vi "Main.vi"() -> ()   [LabVIEW 2017]
uses:
  ExperimentVariables.ctl
  AODControl/AODControlFiles/InterfaceReferences.ctl
  ImageAcquisitionProgram/ImageAcquisitionLibrary/References.ctl
  State.ctl
  SubVIQueues.ctl
  AODControl/MessageQueue/QueueOperations/All Message Queues.ctl
  AODControl/MessageQueue/QueueOperations/Message Cluster.ctl
  CircleControls.ctl
  <vilib>/Utility/error.llb/DialogType.ctl
  AODControl/AODGlobals.vi
  ImageAcquisitionProgram/ImageAcquisitionLibrary/GlobalFrontPanelReferences.vi
  MessageQueue/QueueOperations/Enqueue Message (Single).vi
  AODControl/AODControl.lvlib
  MessageQueue/MessageQueue.lvlib
  AODControl/MessageQueue/MessageQueue.lvlib
  ImageAcquisitionProgram/ImageAcquisitionLibrary/ImageAcquisitionLibrary.lvlib
panel:
  in  "Angle":dbl min=0.0 step=0.1 format="%#_6p"
  in  "Seq":bool
  in  "FlipY":bool
  in  "FlipX":bool
  in  "Phase":dbl step=0.1
  in  "Eccen.":dbl=1.0 min=0.0 step=0.05
  in  "Run":bool
  in  "Abort":bool
  in  "Script Path":path=path "D:/Dropbox/MyPrograms/LabViewLibraries/AODExperimentControls/ReologyScript.vi"
  in  "HexLatt":bool
  in  "Hold":bool
  in  "Hold":bool
  in  "Lattice Constant":dbl=10.0 step=0.05
  in  "Size":i32=1 min=1 step=1
  in  "PointSpec":enum32{"No. Of Points", "Density"}(radio)
  in  "No. of Points":i32=3 step=1
  in  "Exit":bool
  in  "Settings":T1={"Calibration Input"=[], "CalibrationResults"={"Center in Pixels"=[374.0120339529387, 375.46592887074246], "Angle"=0.022945275255000355, "Pixels/MHz X"=0.0, "Pixels/MHz Y"=0.0}, "Highlight"=[], "Running Script"=refnum}
  in  "Density":dbl=1.0 step=0.05
  in  "Center":cluster{"X":dbl, "Y":dbl}
  in  "Radius":dbl=10.0 step=0.05
  in  "Circle":bool
  in  "Exit Button":bool
  in  "Load":bool
  in  "Save":bool
  in  "Reset":bool
  out "Points":i32[][](array[numeric])
  in  "Calibrate":bool
  # "Draw an Ellipse"
  # "Draw a Hexagonal Lattice"
  # "Run a Script"
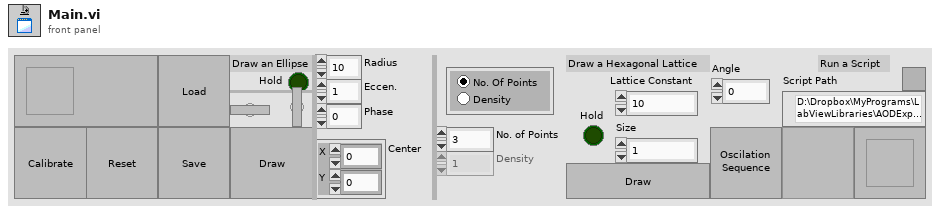
[diagram p1: front panel]
types:
  T1 = typedef "ExperimentVariables.ctl" = cluster{"Calibration Input":i32[][], "CalibrationResults":cluster{"Center in Pixels":dbl[], "Angle":dbl, "Pixels/MHz X":dbl, "Pixels/MHz Y":dbl}, "Highlight":i32[], "Running Script":refnum<vi>}
  T2 = typedef "SubVIQueues.ctl" = cluster{"AOD Queue":T3}
  T3 = typedef "AODControl.lvlib/MessageQueue.lvlib/All Message Queues.ctl" = cluster{" AOD Interface":refnum<queue>}
  T4 = typedef "State.ctl" = enum16{"Point", "Move", "Calibrating"}
  T5 = typedef "ExperimentControls" = cluster{"AOD Controls":T6, "ImageAcquisitionRefs":T7}
  T6 = typedef "AODControl.lvlib/InterfaceReferences.ctl" = cluster{"AOD Points Display":refnum<vi>, "AOD Array":refnum<vi>, "AOD Array Size":refnum<vi>, "Replace Array List":refnum<vi>, "Replace List":refnum<vi>, "Remove":refnum<vi>, "Index":refnum<vi>, "Move":refnum<vi>, "X":refnum<vi>, "Y":refnum<vi>, "Add":refnum<vi>, "Load":refnum<vi>, "Save":refnum<vi>, "Exit":refnum<vi>, "Dynamic":refnum<vi>, "Rotate":refnum<vi>, "Rotation Speed":refnum<vi>, "Scaling Speed":refnum<vi>, "X Trans Speed":refnum<vi>, "Y Trans Speed":refnum<vi>, "Movie Array":refnum<vi>}
  T7 = typedef "ImageAcquisitionLibrary.lvlib/References.ctl" = cluster{"Acquire":refnum<vi>, "Rec":refnum<vi>, "Tracking":refnum<vi>, "Settings":refnum<vi>, "Stop":refnum<vi>, "Initialized?":bool, "ImDisplay":refnum<vi>}
  T8 = typedef "MessageQueue.lvlib/All Message Queues.ctl" = cluster{" Interface":refnum<queue>, "Joystick":refnum<queue>}
  T9 = typedef "CircleControls.ctl" = cluster{"Radius":dbl, "No. of Points":i32, "Center":cluster{"X":dbl, "Y":dbl}, "Circle":bool, "Density":dbl, "PointSpec":enum32{"No. Of Points", "Density"}, "Hold":bool, "Size":i32, "LatC":dbl, "Eccentricity":dbl, "Phase":dbl}
  T10 = enum8{"Enabled", "Disabled", "Disabled and Grayed Out"}
  T11 = typedef "DialogType.ctl" = u16
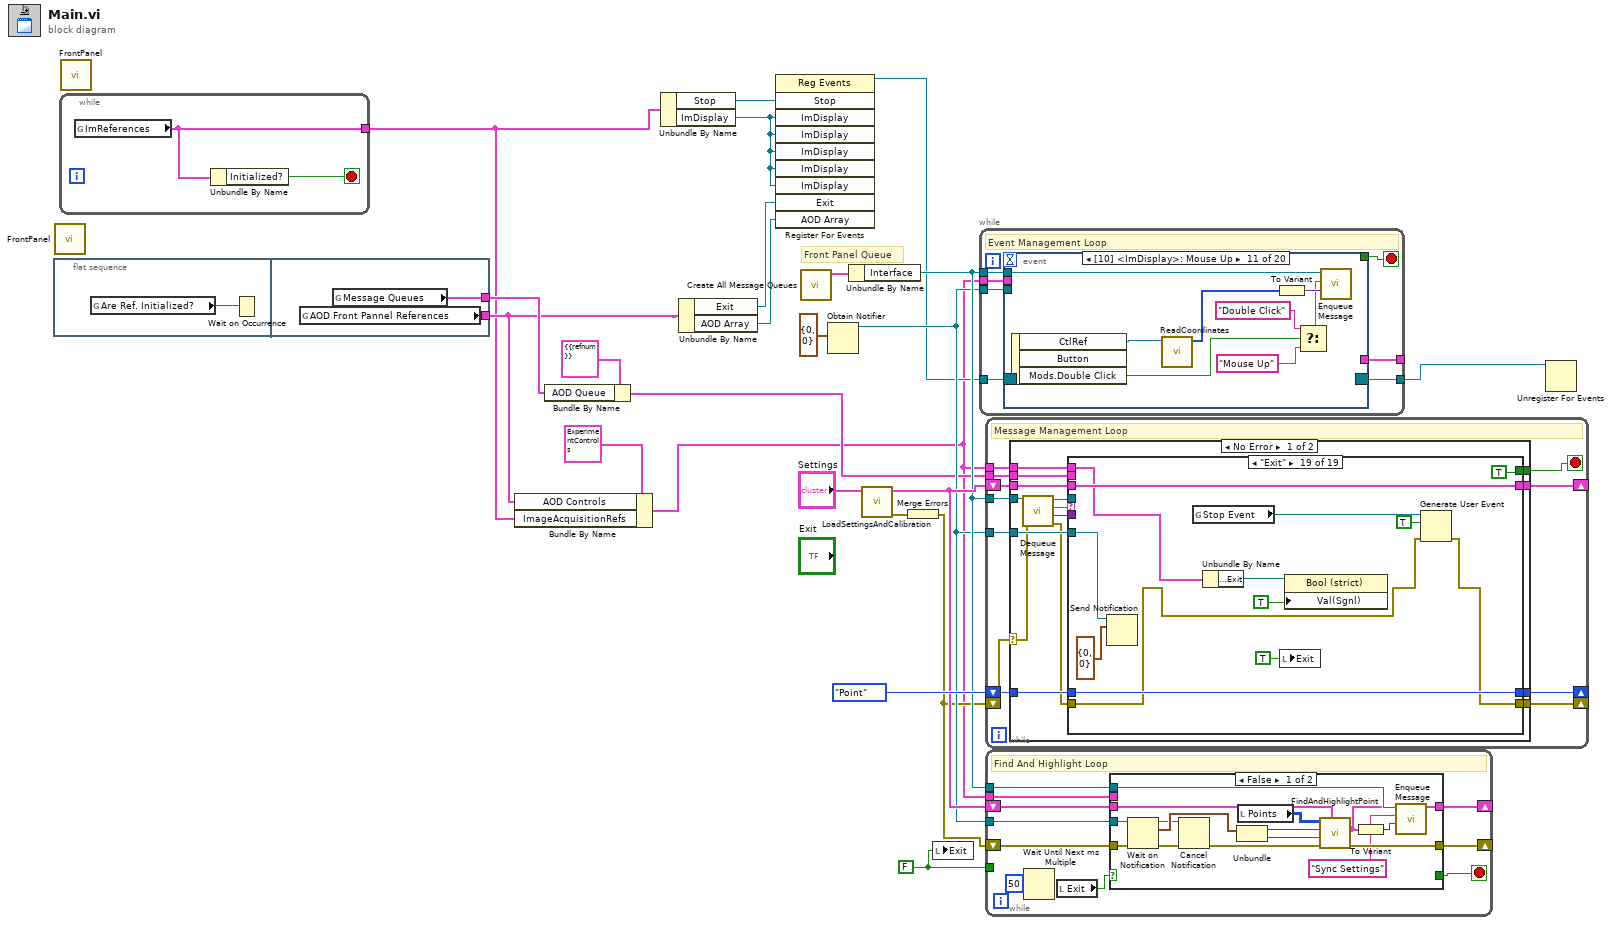
[diagram p0: block diagram]
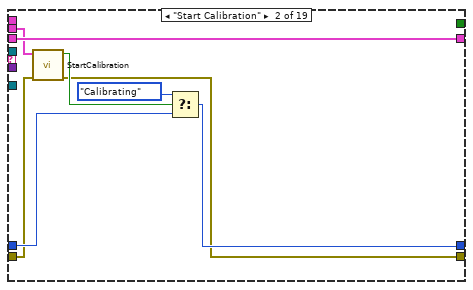
[diagram p4: hidden frame]
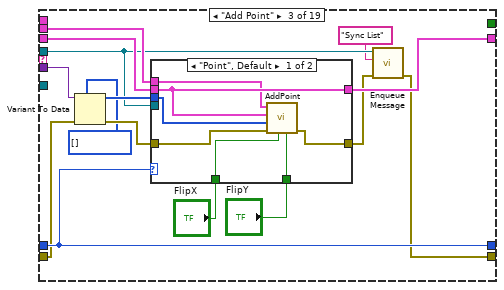
[diagram p5: hidden frame]
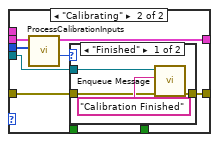
[diagram p6: hidden frame]
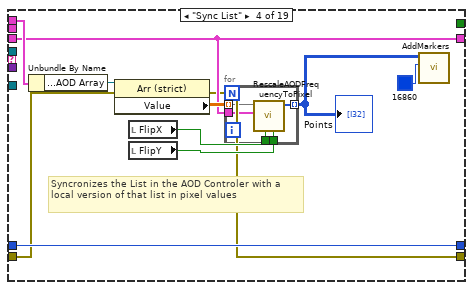
[diagram p8: hidden frame]
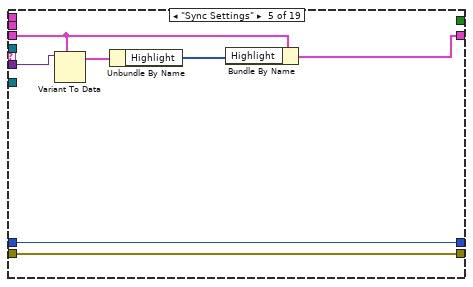
[diagram p9: hidden frame]
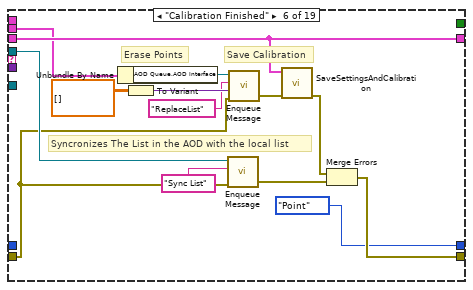
[diagram p10: hidden frame]
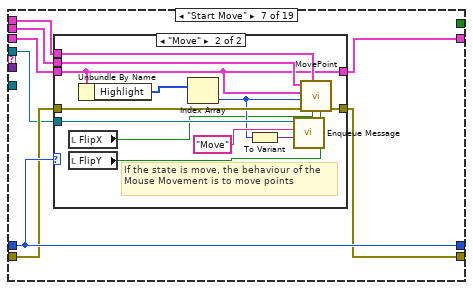
[diagram p11: hidden frame]
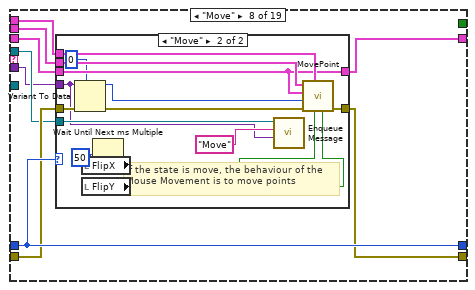
[diagram p13: hidden frame]
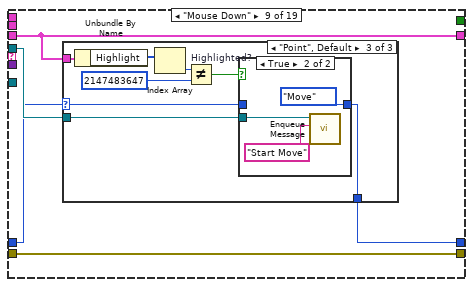
[diagram p15: hidden frame]
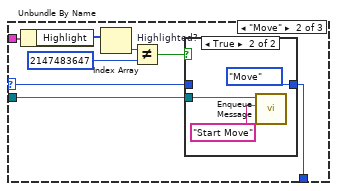
[diagram p17: hidden frame]
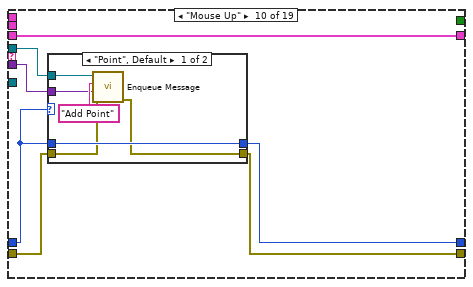
[diagram p20: hidden frame]
diagram:
  w17 = FALSE
  # "Front Panel Queue"
  n1 = flat-sequence {
    tunnel: [w26] -> w9
    tunnel: [w25] -> w6
    frame #0 {
      n2 = global read "AODGlobals.vi" "Are Ref. Initialized?"() -> (w24:refnum<k4>)
      n3 = Wait on Occurrence(2:w24) -> ()  [unwired: 2 in, 1 out]
    }
    frame #1 {
      n4 = global read "AODGlobals.vi" "AOD Front Pannel References"() -> (w25:T6)
      n5 = global read "AODGlobals.vi" "Message Queues"() -> (w26:T3)
    }
  }
  n6 = call "FrontPanel.vi"() -> ()  [unwired: 12 in]
  n7 = while {
    tunnel: [w27] -> w1
    stop <- w28 stop-if-true
    n8 = global read "GlobalFrontPanelReferences.vi" "ImReferences"() -> (w27:T7)
    n9 = Unbundle By Name(w27) -> ("Initialized?"=w28:bool)
  }
  n10 = call "FrontPanel.vi"() -> ()  [unwired: 12 in]
  n11 = Bundle By Name(cluster=T5 {"AOD Controls"={"AOD Points Display"=refnum, "AOD Array"=refnum, "AOD Array Size"=refnum, "Replace Array List"=refnum, "Replace List"=refnum, "Remove"=refnum, "Index"=refnum, "Move"=refnum, "X"=refnum, "Y"=refnum, "Add"=refnum, "Load"=refnum, "Save"=refnum, "Exit"=refnum, "Dynamic"=refnum, "Rotate"=refnum, "Rotation Speed"=refnum, "Scaling Speed"=refnum, "X Trans Speed"=refnum, "Y Trans Speed"=refnum, "Movie Array"=refnum}, "ImageAcquisitionRefs"={"Acquire"=refnum, "Rec"=refnum, "Tracking"=refnum, "Settings"=refnum, "Stop"=refnum, "Initialized?"=FALSE, "ImDisplay"=refnum}}, "AOD Controls"=w6, "ImageAcquisitionRefs"=w1) -> (w4:T5)
  n12 = Bundle By Name(cluster=T2 {"AOD Queue"={" AOD Interface"=refnum}} ("Queues Out"), "AOD Queue"=w9) -> (w10:T2)
  n13 = Unbundle By Name(w1) -> ("Stop"=w3:refnum<vi>, "ImDisplay"=w2:refnum<vi>)
  n14 = Unbundle By Name(w6) -> ("Exit"=w8:refnum<vi>, "AOD Array"=w7:refnum<vi>)
  n15 = register-events(w3, w2, w2, w2, w2, w2, w8, w7) -> (reference out=w12:refnum<event-registration>)  [unwired: 2 in, 1 out]
  n16 = call "Create All Message Queues.vi"() -> ("Message Queues out"=w23:T8)  [unwired: 10 in, 1 out]
  n17 = Obtain Notifier(notification data type=cluster{"X":i32, "Y":i32} {"X"=0, "Y"=0} ("Last Mouse Position:All Elements")) -> (notifier out=w14:refnum<notifier>)  [unwired: 3 in, 2 out]
  n18 = Unbundle By Name(w23) -> ("Interface"=w15:refnum<queue>)
  n19 = call "LoadSettingsAndCalibration.vi"("Cluster in"="Settings") -> ("error out"=w19:errorcluster, "Cluster out"=w16:T1)  [unwired: 9 in]
  n20 = Merge Errors(w19) -> (w13:errorcluster)
  n21 = local write "Exit"(w17) -> ()
  n22 = while {
    tunnel: w12 -> [w35]
    tunnel: w15 -> [w34]
    tunnel: w4 -> [w33]
    tunnel: [w32] -> w21
    tunnel: w14 -> [w30]
    tunnel: [w29] -> _
    stop <- w31 stop-if-true
    # "Event Management Loop"
    n23 = event shown="[10] <ImDisplay>: Mouse Up" {
      selector: w35 -> [_ _ _ _ _ _ _ _ _ _ _ _ w95 w96 _ _ _ _ _ _]
      dyn-events: [_ _ _ _ _ _ _ _ _ _ _ _ w94 w99 _ _ _ _ _ _] -> w32
      timeout: _ -> [_ _ _ _ _ _ _ _ _ _ _ _ _ _ _ _ _ _ _ _]
      tunnel: w34 -> [w36 w39 w43 w45 w47 w49 w63 w72 _ w81 w89 w91 _ _ _ w104 w107 w109 w111 w114]
      tunnel: w33 -> [_ _ _ _ _ _ _ _ _ _ _ _ w93 w98 _ _ _ _ _ _]
      tunnel: [TRUE TRUE _ _ _ _ _ _ _ _ _ _ _ _ _ _ _ _ TRUE TRUE] -> w31
      tunnel: w30 -> [_ _ _ _ _ _ _ _ _ _ _ _ _ _ w101 _ _ _ _ _]
      tunnel: [_ _ _ _ _ _ w60 w69 _ _ _ _ _ _ _ _ _ _ _ _] -> w29
      event Value Change {
        n24 = event-data() -> ()  [unwired: 1 in, 1 out]
        n25 = call-poly "Enqueue Message.vi"("Message"="Exit", "Message Queue"=w36) -> ()  [unwired: 8 in, 2 out]
      }
      event Value Change {
        n26 = event-data() -> ()  [unwired: 1 in, 1 out]
        n27 = call-poly "Enqueue Message.vi"("Message"="Exit", "Message Queue"=w39) -> ()  [unwired: 8 in, 2 out]
      }
      event "Calibrate": Value Change {
        n28 = event-data() -> ()  [unwired: 1 in, 1 out]
        n29 = call-poly "Enqueue Message.vi"("Message"="Start Calibration", "Message Queue"=w43) -> ()  [unwired: 8 in, 2 out]
      }
      event "Reset": Value Change {
        n30 = event-data() -> ()  [unwired: 1 in, 1 out]
        n31 = call-poly "Enqueue Message.vi"("Message"="Reset AOD", "Message Queue"=w45) -> ()  [unwired: 8 in, 2 out]
      }
      event "Save": Value Change {
        n32 = event-data() -> ()  [unwired: 1 in, 1 out]
        n33 = call-poly "Enqueue Message.vi"("Message"="Save List", "Message Queue"=w47) -> ()  [unwired: 8 in, 2 out]
      }
      event "Load": Value Change {
        n34 = event-data() -> ()  [unwired: 1 in, 1 out]
        n35 = call-poly "Enqueue Message.vi"("Message"="Load List", "Message Queue"=w49) -> ()  [unwired: 8 in, 2 out]
      }
      event "Circle", "Center", "Density", "Radius", "No. of Points", "Eccen.", "Phase": Value Change {
        n36 = event-data() -> ()  [unwired: 1 in, 1 out]
        n37 = Bundle(cluster=T9 {"Radius"=0.0, "No. of Points"=0, "Center"={"X"=0.0, "Y"=0.0}, "Circle"=FALSE, "Density"=0.0, "PointSpec"=enum."No. Of Points", "Hold"=FALSE, "Size"=1, "LatC"=10.0, "Eccentricity"=0.0, "Phase"=0.0} ("Cluster"), "Radius"="Radius", "No. of Points"="No. of Points", "Center"="Center", "Circle"="Circle", "Density"="Density", "PointSpec"="PointSpec", "Hold"="Hold", "Eccentricity"="Eccen.", "Phase"="Phase") -> (w60:T9)  [unwired: 2 in]
        n38 = To Variant(anything=w60) -> (Variant=w61:variant)
        n39 = call-poly "Enqueue Message.vi"("Message Data"=w61, "Message"="Circle", "Message Queue"=w63) -> ()  [unwired: 7 in, 2 out]
      }
      event "Size", "Lattice Constant", "HexLatt": Value Change {
        n40 = event-data() -> ()  [unwired: 1 in, 1 out]
        n41 = Bundle By Name(cluster=T9 {"Radius"=0.0, "No. of Points"=0, "Center"={"X"=0.0, "Y"=0.0}, "Circle"=FALSE, "Density"=0.0, "PointSpec"=enum."No. Of Points", "Hold"=FALSE, "Size"=1, "LatC"=10.0, "Eccentricity"=0.0, "Phase"=0.0} ("Cluster"), "Circle"="HexLatt", "LatC"="Lattice Constant", "Size"="Size", "Hold"="Hold") -> (w69:T9)
        n42 = To Variant(anything=w69) -> (Variant=w70:variant)
        n43 = call-poly "Enqueue Message.vi"("Message Data"=w70, "Message"="HexLattice", "Message Queue"=w72) -> ()  [unwired: 7 in, 2 out]
      }
      event "PointSpec": Value Change {
        n44 = event-data() -> ()  [unwired: 1 in, 1 out]
        n45 = local read "PointSpec"() -> (w73:enum32{"No. Of Points", "Density"})
        n46 = case shown="\"No. Of Points\", Default" w73 {
          frame "Density" {
            n47 = property on="No. of Points" class="DigNum (strict)"("DisabledEnum"=T10."Disabled and Grayed Out" ("Disabled")) -> ()  [unwired: 2 in, 2 out]
            n48 = property on="Density" class="DigNum (strict)"("DisabledEnum"=T10."Enabled" ("Disabled")) -> ()  [unwired: 2 in, 2 out]
          }
          frame "No. Of Points", Default {
            n49 = property on="No. of Points" class="DigNum (strict)"("DisabledEnum"=T10."Enabled" ("Disabled")) -> ()  [unwired: 2 in, 2 out]
            n50 = property on="Density" class="DigNum (strict)"("DisabledEnum"=T10."Disabled and Grayed Out" ("Disabled")) -> ()  [unwired: 2 in, 2 out]
          }
        }
      }
      event "Seq": Value Change {
        n51 = event-data() -> ()  [unwired: 1 in, 1 out]
        n52 = To Variant(anything="Angle") -> (Variant=w79:variant)
        n53 = call-poly "Enqueue Message.vi"("Message Data"=w79, "Message"="Program Sequence", "Message Queue"=w81) -> ()  [unwired: 7 in, 2 out]
      }
      event Mouse Up {
        n54 = event-data() -> ("CtlRef"=w86:refnum<vi>, "Mods.Double Click"=w83:bool)  [unwired: 1 in, 1 out]
        n55 = call "ReadCoordinates.vi"("Ctl Refnum"=w86) -> ("appended array"=w87:i32[])  [unwired: 10 in]
        n56 = To Variant(anything=w87) -> (Variant=w88:variant)
        n57 = Select(t="Double Click" ("Message"), s=w83, f="Mouse Up" ("Message")) -> (s? t:f=w82:string)
        n58 = call-poly "Enqueue Message.vi"("Message Data"=w88, "Message"=w82, "Message Queue"=w89) -> ()  [unwired: 7 in, 2 out]
      }
      event Mouse Down {
        n59 = event-data() -> ()  [unwired: 1 in, 3 out]
        n60 = call-poly "Enqueue Message.vi"("Message"="Mouse Down", "Message Queue"=w91) -> ()  [unwired: 8 in, 2 out]
      }
      event Mouse Enter {
        n61 = event-data() -> ()  [unwired: 1 in, 3 out]
        n62 = call "MouseMoveTrackingSwitch.vi"("State"=enum16{"Stop", "Start"}."Start", "Controls Reference In"=w93, "Event Registration Refnum In"=w95) -> ("Event Registration Refnum Out"=w94:refnum<event-registration>)  [unwired: 8 in]
      }
      event Mouse Leave {
        n63 = event-data() -> ()  [unwired: 1 in, 3 out]
        n64 = call "MouseMoveTrackingSwitch.vi"("State"=enum16{"Stop", "Start"}."Stop", "Controls Reference In"=w98, "Event Registration Refnum In"=w96) -> ("Event Registration Refnum Out"=w99:refnum<event-registration>)  [unwired: 8 in]
      }
      event Mouse Move {
        n65 = event-data() -> ("CtlRef"=w102:refnum<vi>)  [unwired: 1 in]
        n66 = property class="ImageControl"(reference=w102) -> ("Last Mouse Position"=w100:cluster{"X":i32, "Y":i32})  [unwired: 1 in, 2 out]
        n67 = Send Notification(notification=w100, notifier=w101) -> ()  [unwired: 1 in, 2 out]
      }
      event Value Change {
        n68 = event-data() -> ()  [unwired: 1 in, 1 out]
        n69 = call-poly "Enqueue Message.vi"("Message"="Sync List", "Message Queue"=w104) -> ()  [unwired: 8 in, 2 out]
      }
      event "Run": Value Change {
        n70 = event-data() -> ()  [unwired: 1 in, 2 out]
        n71 = To Variant(anything="Script Path") -> (Variant=w106:variant)
        n72 = call-poly "Enqueue Message.vi"("Message Data"=w106, "Message"="Run Script", "Message Queue"=w107) -> ()  [unwired: 7 in, 2 out]
      }
      event "Abort": Value Change {
        n73 = event-data() -> ()  [unwired: 1 in, 2 out]
        n74 = call-poly "Enqueue Message.vi"("Message"="Abort Script", "Message Queue"=w109) -> ()  [unwired: 8 in, 2 out]
      }
      event Panel Close {
        n75 = event-data() -> ()  [unwired: 1 in, 1 out]
        n76 = call-poly "Enqueue Message.vi"("Message"="Exit", "Message Queue"=w111) -> ()  [unwired: 8 in, 2 out]
      }
      event "Exit Button": Value Change {
        n77 = event-data() -> ()  [unwired: 1 in, 1 out]
        n78 = call-poly "Enqueue Message.vi"("Message"="Exit", "Message Queue"=w114) -> ()  [unwired: 8 in, 2 out]
      }
    }
  }
  n79 = while {
    tunnel: w15 -> [w117]
    tunnel: w4 -> [w127]
    shift-right: [w125] -> _
    shift-left: w16 -> [w126]
    tunnel: w10 -> [w123]
    shift-right: [w121] -> _
    shift-left: State."Point" ("State") -> [w122]
    shift-right: [w120] -> _
    shift-left: w13 -> [w119]
    tunnel: w14 -> [w118]
    stop <- w124 stop-if-true
    # "Message Management Loop"
    n80 = case shown="No Error" w119 {
      selector: w119 -> [w129 w465]
      tunnel: w127 -> [w142 _]
      tunnel: w126 -> [w141 w470]
      tunnel: [w140 w470] -> w125
      tunnel: [w139 _] -> w124
      tunnel: w123 -> [w138 _]
      tunnel: w122 -> [w135 w469]
      tunnel: [w137 w469] -> w121
      tunnel: [w134 w466] -> w120
      tunnel: w118 -> [w136 _]
      tunnel: w117 -> [w133 _]
      frame No Error {
        n81 = call "Dequeue Message.vi"("error in (no error)"=w129, "Message Queue"=w133) -> ("error out"=w128:errorcluster, "Message Data"=w130:variant, "Message"=w131:string, "dup Message Queue"=w132:refnum<queue>)  [unwired: 6 in]
        n82 = case shown="\"Exit\"" w131 {
          tunnel: w132 -> [_ _ w163 _ _ w218 w225 w248 w273 w308 w326 _ _ _ _ _ _ _ _]
          tunnel: w130 -> [_ _ w168 _ w210 _ _ w247 _ w307 _ _ _ _ w365 w420 w431 _ _]
          tunnel: w142 -> [_ _ _ w198 _ _ w230 w253 _ _ _ _ _ _ _ _ _ _ w461]
          tunnel: w141 -> [w145 w153 w166 w195 w207 w224 w232 w255 w276 w304 w323 w338 w345 w352 w369 w423 w435 w451 w464]
          tunnel: [w145 w153 w165 w195 w204 w224 w231 w254 w276 w304 w323 w338 w345 w352 w369 w423 w435 w451 w464] -> w140
          tunnel: [_ _ _ _ _ _ _ _ _ _ _ _ _ _ _ _ _ _ TRUE] -> w139
          tunnel: w138 -> [_ w152 w164 _ _ w219 w228 w251 _ _ w329 w336 w343 w350 w367 w421 w433 _ _]
          tunnel: w128 -> [w143 w147 w159 w193 w208 w215 w227 w250 w274 w303 w321 w333 w340 w347 w366 w419 w432 w449 w454]
          tunnel: [w144 w149 w161 w194 w209 State."Point" ("State") w229 w252 w275 w305 w324 w337 w344 w351 w368 w401 w434 w450 w462] -> w137
          tunnel: w136 -> [_ _ _ _ _ _ _ _ _ _ _ _ _ _ _ _ _ _ w460]
          tunnel: w135 -> [w144 w151 w161 w194 w209 _ w229 w252 w272 w306 w325 w337 w344 w351 w368 w401 w434 w450 w462]
          tunnel: [w143 w146 w157 w190 w208 w212 w226 w249 w274 w302 w322 w332 w339 w346 w363 w402 w429 w449 w453] -> w134
          frame "Initialize" {
          }
          frame "Start Calibration" {
            n83 = call "StartCalibration.vi"("error in"=w147, "Queues Cluster"=w152) -> ("error out"=w146:errorcluster, "Started?"=w150:bool)  [unwired: 4 in]
            n84 = Select(t=State."Calibrating" ("State"), s=w150, f=w151) -> (s? t:f=w149:T4)
          }
          frame "Add Point" {
            n85 = Variant To Data(error in=w159, type=i32[] [] ("appended array"), Variant=w168) -> (data=w167:i32[], error out=w160:errorcluster)
            n86 = case shown="\"Point\", Default" w161 {
              tunnel: w167 -> [w175 w182]
              tunnel: w166 -> [w174 w181]
              tunnel: [w174 w180] -> w165
              tunnel: w163 -> [_ w179]
              tunnel: w164 -> [w171 _]
              tunnel: w160 -> [w172 w177]
              tunnel: [w173 w176] -> w158
              tunnel: "FlipY" -> [w170 _]
              tunnel: "FlipX" -> [w169 _]
              frame "Point", Default {
                n87 = call "AddPoint.vi"("FlipY"=w170, "FlipX"=w169, "error in (no error)"=w172, "Pixels"=w175, 10:w174, "Cluster"=w171) -> ("error out"=w173:errorcluster)  [unwired: 5 in]
              }
              frame "Calibrating" {
                n88 = call "ProcessCalibrationInputs.vi"("Point"=w182, "ExperimentVariables"=w181) -> ("Status"=w178:enum16{"Finished", "Waiting"}, "output cluster"=w180:T1)  [unwired: 8 in]
                n89 = case shown="\"Finished\"" w178 {
                  tunnel: w179 -> [w186 _]
                  tunnel: w177 -> [w184 w187]
                  tunnel: [w183 w187] -> w176
                  frame "Finished" {
                    n90 = call-poly "Enqueue Message.vi"("error in (no error)"=w184, "Message"="Calibration Finished", "Message Queue"=w186) -> ("error out"=w183:errorcluster)  [unwired: 7 in, 1 out]
                  }
                  frame "Waiting", Default {
                  }
                }
              }
            }
            n91 = call-poly "Enqueue Message.vi"("error in (no error)"=w158, "Message"="Sync List", "Message Queue"=w163) -> ("error out"=w157:errorcluster)  [unwired: 7 in, 1 out]
          }
          frame "Sync List" {
            # "Syncronizes the List in the AOD Controler with a local version of that list in pixel values"
            n92 = Unbundle By Name(w198) -> ("AOD Controls.AOD Array"=w197:refnum<vi>)
            n93 = property class="Arr (strict)"(reference=w197, error in=w193) -> (error out=w190:errorcluster, "Value"=w196:dbl[][])  [unwired: 1 out]
            n94 = local read "FlipX"() -> (w192:bool)
            n95 = local read "FlipY"() -> (w191:bool)
            n96 = for {
              tunnel: w196 -> [w203] mode=indexing
              tunnel: [w202] -> w188 mode=indexing
              tunnel: w195 -> [w201]
              tunnel: w192 -> [w200]
              tunnel: w191 -> [w199]
              n97 = call "RescaleAODFrequencyToPixel.vi"("FlipY 2"=w199, "FlipX 2"=w200, 10:w201, "Array 2"=w203) -> ("Pixels 2"=w202:i32[])  [unwired: 7 in]
            }
            "Points" <- w188
            n98 = call "AddMarkers.vi"("Color"=u32 16860, "Pixels 3"=w188) -> ()  [unwired: 10 in]
          }
          frame "Sync Settings" {
            n99 = Variant To Data(type=w207, Variant=w210) -> (data=w206:T1)  [unwired: 1 in, 1 out]
            n100 = Unbundle By Name(w206) -> ("Highlight"=w205:i32[])
            n101 = Bundle By Name(cluster=w207, "Highlight"=w205) -> (w204:T1)
          }
          frame "Calibration Finished" {
            # "Syncronizes The List in the AOD with the local list"
            # "Erase Points"
            # "Save Calibration"
            n102 = Unbundle By Name(w219) -> ("AOD Queue.AOD Interface"=w220:refnum<queue>)
            n103 = To Variant(anything=dbl[][] [] ("Array")) -> (Variant=w223:variant)
            n104 = call-poly "Enqueue Message.vi"("error in (no error)"=w215, "Message"="Sync List", "Message Queue"=w218) -> ("error out"=w213:errorcluster)  [unwired: 7 in, 1 out]
            n105 = call-poly "Enqueue Message.vi"("error in (no error)"=w215, "Message Data"=w223, "Message"="ReplaceList", "Message Queue"=w220) -> ("error out"=w216:errorcluster)  [unwired: 6 in, 1 out]
            n106 = call "SaveSettingsAndCalibration.vi"("error in (no error)"=w216, "Cluster"=w224) -> ("error out"=w214:errorcluster)  [unwired: 9 in]
            n107 = Merge Errors(w214, w213) -> (w212:errorcluster)
          }
          frame "Start Move" {
            n108 = case shown="\"Move\"" w229 {
              tunnel: w232 -> [w234 w240]
              tunnel: [w234 w240] -> w231
              tunnel: w230 -> [_ w246]
              tunnel: w228 -> [_ w245]
              tunnel: w227 -> [w233 w244]
              tunnel: [w233 w243] -> w226
              tunnel: w225 -> [_ w241]
              frame "Point", Default {
                # "If the state is point, the behaviour of the \nMouse Movement is to highlight points"
              }
              frame "Move" {
                # "If the state is move, the behaviour of the \nMouse Movement is to move points"
                n109 = local read "FlipX"() -> (w236:bool)
                n110 = local read "FlipY"() -> (w235:bool)
                n111 = Unbundle By Name(w240) -> ("Highlight"=w239:i32[])
                n112 = Index Array(array=w239) -> (element=w237:i32)  [unwired: 1 in]
                n113 = To Variant(anything=w237) -> (Variant=w238:variant)
                n114 = call-poly "Enqueue Message.vi"("Message Data"=w238, "Message"="Move", "Message Queue"=w241) -> ()  [unwired: 7 in, 2 out]
                n115 = call "MovePoint.vi"("FlipY"=w235, "FlipX"=w236, "Controls Reference Out"=w246, "error in (no error)"=w244, "Index"=w237, "Settings In"=w240, "Queues Out"=w245) -> ("error out"=w243:errorcluster)  [unwired: 4 in]
              }
            }
          }
          frame "Move" {
            n116 = case shown="\"Move\"" w252 {
              tunnel: w255 -> [w257 w266]
              tunnel: [w257 w266] -> w254
              tunnel: w253 -> [_ w271]
              tunnel: w251 -> [_ w270]
              tunnel: w250 -> [w256 w263]
              tunnel: [w256 w269] -> w249
              tunnel: w248 -> [_ w267]
              tunnel: w247 -> [_ w261]
              frame "Point", Default {
                # "If the state is point, the behaviour of the \nMouse Movement is to highlight points"
              }
              frame "Move" {
                # "If the state is move, the behaviour of the \nMouse Movement is to move points"
                n117 = Variant To Data(error in=w263, type=0 ("Index"), Variant=w261) -> (data=w264:i32, error out=w262:errorcluster)
                n118 = local read "FlipX"() -> (w259:bool)
                n119 = local read "FlipY"() -> (w258:bool)
                n120 = Wait Until Next ms Multiple(millisecond multiple=u32 50) -> ()  [unwired: 1 out]
                n121 = call-poly "Enqueue Message.vi"("Message Data"=w261, "Message"="Move", "Message Queue"=w267) -> ()  [unwired: 7 in, 2 out]
                n122 = call "MovePoint.vi"("FlipY"=w258, "FlipX"=w259, "Controls Reference Out"=w271, "error in (no error)"=w262, "Index"=w264, "Settings In"=w266, "Queues Out"=w270) -> ("error out"=w269:errorcluster)  [unwired: 4 in]
              }
            }
          }
          frame "Mouse Down" {
            n123 = case shown="\"Point\", Default" w272 {
              selector: w272 -> [w277 w278 w290]
              tunnel: w276 -> [_ w284 w296]
              tunnel: [w277 w280 w292] -> w275
              tunnel: w273 -> [_ w279 w291]
              frame "Calibrating" {
              }
              frame "Move" {
                n124 = Unbundle By Name(w284) -> ("Highlight"=w283:i32[])
                n125 = Index Array(array=w283) -> (element=w282:i32)  [unwired: 1 in]
                n126 = Not Equal? "Highlighted?"(x=w282, y=2147483647) -> (x != y?=w281:bool)
                n127 = case shown="True" w281 {
                  tunnel: [w286 State."Move" ("State")] -> w280
                  tunnel: w278 -> [w286 _]
                  tunnel: w279 -> [_ w287]
                  frame False {
                  }
                  frame True {
                    n128 = call-poly "Enqueue Message.vi"("Message"="Start Move", "Message Queue"=w287) -> ()  [unwired: 8 in, 2 out]
                  }
                }
              }
              frame "Point", Default {
                n129 = Unbundle By Name(w296) -> ("Highlight"=w295:i32[])
                n130 = Index Array(array=w295) -> (element=w294:i32)  [unwired: 1 in]
                n131 = Not Equal? "Highlighted?"(x=w294, y=2147483647) -> (x != y?=w293:bool)
                n132 = case shown="True" w293 {
                  tunnel: [w298 State."Move" ("State")] -> w292
                  tunnel: w290 -> [w298 _]
                  tunnel: w291 -> [_ w299]
                  frame False {
                  }
                  frame True {
                    n133 = call-poly "Enqueue Message.vi"("Message"="Start Move", "Message Queue"=w299) -> ()  [unwired: 8 in, 2 out]
                  }
                }
              }
            }
          }
          frame "Mouse Up" {
            n134 = case shown="\"Point\", Default" w306 {
              tunnel: w308 -> [w314 w316]
              tunnel: w307 -> [w312 _]
              tunnel: w306 -> [w311 _]
              tunnel: [w311 State."Point" ("State")] -> w305
              tunnel: w303 -> [w310 w318]
              tunnel: [w309 w317] -> w302
              frame "Point", Default {
                n135 = call-poly "Enqueue Message.vi"("error in (no error)"=w310, "Message Data"=w312, "Message"="Add Point", "Message Queue"=w314) -> ("error out"=w309:errorcluster)  [unwired: 6 in, 1 out]
              }
              frame "Move" {
                n136 = Flush Queue(queue=w316) -> (queue out=w315:refnum<queue>)  [unwired: 1 in, 2 out]
                n137 = call-poly "Enqueue Message.vi"("error in (no error)"=w318, "Message"="Sync List", "Message Queue"=w315) -> ("error out"=w317:errorcluster)  [unwired: 7 in, 1 out]
              }
            }
          }
          frame "Double Click" {
            n138 = call "DeletePoint.vi"("error in"=w321, "Cluster in"=w323, "Queues Input"=w329) -> ("error out"=w327:errorcluster)  [unwired: 8 in]
            n139 = case shown="\"Move\"" w325 {
              tunnel: w325 -> [w330 _]
              tunnel: [w330 State."Point" ("State")] -> w324
              frame "Point", Default {
              }
              frame "Move" {
              }
            }
            n140 = call-poly "Enqueue Message.vi"("error in (no error)"=w327, "Message"="Sync List", "Message Queue"=w326) -> ("error out"=w322:errorcluster)  [unwired: 7 in, 1 out]
          }
          frame "Reset AOD" {
            n141 = Unbundle By Name(w336) -> ("AOD Queue.AOD Interface"=w335:refnum<queue>)
            n142 = call-poly "Enqueue Message.vi"("error in (no error)"=w333, "Message"="ResetList", "Message Queue"=w335) -> ("error out"=w332:errorcluster)  [unwired: 7 in, 1 out]
          }
          frame "Save List" {
            n143 = Unbundle By Name(w343) -> ("AOD Queue.AOD Interface"=w342:refnum<queue>)
            n144 = call-poly "Enqueue Message.vi"("error in (no error)"=w340, "Message"="SaveList", "Message Queue"=w342) -> ("error out"=w339:errorcluster)  [unwired: 7 in, 1 out]
          }
          frame "Load List" {
            n145 = Unbundle By Name(w350) -> ("AOD Queue.AOD Interface"=w349:refnum<queue>)
            n146 = call-poly "Enqueue Message.vi"("error in (no error)"=w347, "Message"="LoadList", "Message Queue"=w349) -> ("error out"=w346:errorcluster)  [unwired: 7 in, 1 out]
          }
          frame "Circle" {
            n147 = Variant To Data(type=T9 {"Radius"=0.0, "No. of Points"=0, "Center"={"X"=0.0, "Y"=0.0}, "Circle"=FALSE, "Density"=0.0, "PointSpec"=enum."No. Of Points", "Hold"=FALSE, "Size"=1, "LatC"=10.0, "Eccentricity"=0.0, "Phase"=0.0} ("Cluster"), Variant=w365) -> (data=w364:T9)  [unwired: 1 in, 1 out]
            n148 = Unbundle By Name(w364) -> ("Center"=w357:cluster{"X":dbl, "Y":dbl}, "Radius"=w358:dbl, "No. of Points"=w359:i32, "Circle"=w356:bool, "Density"=w360:dbl, "PointSpec"=w361:enum32{"No. Of Points", "Density"}, "Hold"=w355:bool, "Eccentricity"=w354:dbl, "Phase"=w353:dbl)
            n149 = case shown="True" w356 {
              tunnel: w367 -> [_ w388]
              tunnel: w366 -> [w370 w386]
              tunnel: [w370 w383] -> w363
              tunnel: w361 -> [_ w382]
              tunnel: w360 -> [_ w381]
              tunnel: w359 -> [_ w380]
              tunnel: w358 -> [_ w378]
              tunnel: w357 -> [_ w377]
              tunnel: w355 -> [_ w374]
              tunnel: w354 -> [_ w372]
              tunnel: w353 -> [_ w371]
              frame False {
              }
              frame True {
                n150 = case shown="\"Density\"" w382 {
                  tunnel: w381 -> [_ w397]
                  tunnel: w378 -> [w391 w396]
                  tunnel: w380 -> [w389 _]
                  tunnel: [w389 w395] -> w379
                  frame "No. Of Points", Default {
                    n151 = Multiply(x=w391, y=6.283185307179586) -> (x*y=w393:dbl)
                    n152 = To Double Precision Float(number=w389) -> (double precision float=w390:dbl)
                    n153 = Divide(x=w390, y=w393) -> (x/y=w394:dbl)
                    n154 = local write "Density"(w394) -> ()
                  }
                  frame "Density" {
                    n155 = Compound Arithmetic op=MULTIPLY(w396, w397, 6.283185307179586) -> (w399:dbl)
                    n156 = Round To Nearest(number=w399) -> (nearest integer value=w400:dbl)
                    n157 = To Long Integer(number=w400) -> (32bit integer=w395:i32)
                    n158 = local write "No. of Points"(w395) -> ()
                  }
                }
                n159 = Unbundle By Name(w388) -> ("AOD Queue.AOD Interface"=w387:refnum<queue>)
                n160 = Select(t="AddPoints" ("Message"), s=w374, f="ReplaceList" ("Message")) -> (s? t:f=w373:string)
                n161 = call "DrawCircle.vi"("Phase"=w371, "Eccentricity"=w372, "No Of Points"=w379, "Radius"=w378, "Center"=w377) -> ("Array"=w384:dbl[][])  [unwired: 6 in]
                n162 = To Variant(anything=w384) -> (Variant=w385:variant)
                n163 = call-poly "Enqueue Message.vi"("error in (no error)"=w386, "Message Data"=w385, "Message"=w373, "Message Queue"=w387) -> ("error out"=w383:errorcluster)  [unwired: 6 in, 1 out]
              }
            }
          }
          frame "Program Sequence" {
            n164 = Variant To Data(error in=w419, type=0.0, Variant=w420) -> (data=w406:dbl, error out=w402:errorcluster)
            n165 = local read "No. of Points"() -> (w417:i32)
            n166 = local read "PointSpec"() -> (w413:enum32{"No. Of Points", "Density"})
            n167 = local read "Density"() -> (w414:dbl)
            n168 = local read "Radius"() -> (w418:dbl)
            n169 = local read "Center"() -> (w416:cluster{"X":dbl, "Y":dbl})
            n170 = local read "Eccen."() -> (w411:dbl)
            n171 = local read "Phase"() -> (w410:dbl)
            n172 = local read "Circle"() -> (w415:bool)
            n173 = local read "Hold"() -> (w412:bool)
            n174 = Bundle By Name(cluster=T9 {"Radius"=0.0, "No. of Points"=0, "Center"={"X"=0.0, "Y"=0.0}, "Circle"=FALSE, "Density"=0.0, "PointSpec"=enum."No. Of Points", "Hold"=FALSE, "Size"=1, "LatC"=10.0, "Eccentricity"=0.0, "Phase"=0.0} ("Cluster"), "Radius"=w418, "No. of Points"=w417, "Center"=w416, "Circle"=w415, "Density"=w414, "PointSpec"=w413, "Hold"=w412, "Eccentricity"=w411, "Phase"=w410) -> (w409:T9)
            n175 = Unbundle By Name(w421) -> ("AOD Queue.AOD Interface"=w422:refnum<queue>)
            n176 = call "ProgramSequence.vi"("Angle"=w406, "Cluster"=w409) -> ("Sequence"=w405:dbl[][][])  [unwired: 9 in]
            n177 = To Variant(anything=w405) -> (Variant=w404:variant)
            n178 = call-poly "Enqueue Message.vi"("Message Data"=w404, "Message"="ReplaceSequence", "Message Queue"=w422) -> ()  [unwired: 7 in, 2 out]
          }
          frame "HexLattice" {
            n179 = Variant To Data(type=T9 {"Radius"=0.0, "No. of Points"=0, "Center"={"X"=0.0, "Y"=0.0}, "Circle"=FALSE, "Density"=0.0, "PointSpec"=enum."No. Of Points", "Hold"=FALSE, "Size"=1, "LatC"=10.0, "Eccentricity"=0.0, "Phase"=0.0} ("Cluster"), Variant=w431) -> (data=w430:T9)  [unwired: 1 in, 1 out]
            n180 = Unbundle By Name(w430) -> ("LatC"=w425:dbl, "Size"=w426:i32, "Circle"=w424:bool, "Hold"=w427:bool)
            n181 = case shown="True" w424 {
              tunnel: w433 -> [_ w448]
              tunnel: w432 -> [w436 w446]
              tunnel: [w436 w444] -> w429
              tunnel: w427 -> [_ w437]
              tunnel: w426 -> [_ w442]
              tunnel: w425 -> [_ w443]
              frame False {
              }
              frame True {
                n182 = Unbundle By Name(w448) -> ("AOD Queue.AOD Interface"=w447:refnum<queue>)
                n183 = Select(t="AddPoints" ("Message"), s=w437, f="ReplaceList" ("Message")) -> (s? t:f=w438:string)
                n184 = call "DrawHexagonalLattice.vi"("Size"=w442, "Lattice Constant"=w443) -> ("E1"=w441:dbl[][])  [unwired: 9 in]
                n185 = To Variant(anything=w441) -> (Variant=w445:variant)
                n186 = call-poly "Enqueue Message.vi"("error in (no error)"=w446, "Message Data"=w445, "Message"=w438, "Message Queue"=w447) -> ("error out"=w444:errorcluster)  [unwired: 6 in, 1 out]
              }
            }
          }
          frame Default {
          }
          frame "Exit" {
            n187 = Send Notification(notification=cluster{"X":i32, "Y":i32} {"X"=0, "Y"=0} ("Last Mouse Position:All Elements"), notifier=w460) -> ()  [unwired: 1 in, 2 out]
            n188 = global read "GlobalFrontPanelReferences.vi" "Stop Event"() -> (w455:refnum<user-event>)
            n189 = Unbundle By Name(w461) -> ("AOD Controls.Exit"=w458:refnum<vi>)
            n190 = local write "Exit"(TRUE ("Exit")) -> ()
            n191 = property class="Bool (strict)"(reference=w458, "Val(Sgnl)"=TRUE) -> ()  [unwired: 1 in, 2 out]
            n192 = Generate User Event(user event=w455, event data cluster=TRUE ("event data"), error in=w454) -> (error out=w453:errorcluster)  [unwired: 1 in, 1 out]
          }
        }
      }
      frame Error {
        w467 = T11 2 items=["no dialog", "OK message", "continue or stop message", "OK message + warnings", "continue/stop + warnings"] ("type of dialog (OK msg:1)")
        n193 = call <vilib>:"Simple Error Handler.vi"("type of dialog (OK msg:1)"=w467, "error in (no error)"=w465) -> ("error out"=w468:errorcluster)  [unwired: 3 in, 4 out]
        n194 = call <vilib>:"Clear Errors.vi"("error in (no error)"=w468) -> ("error out"=w466:errorcluster)  [unwired: 5 in, 1 out]
      }
    }
  }
  n195 = while {
    tunnel: w14 -> [w480]
    tunnel: w4 -> [w473]
    shift-right: [w479] -> _
    shift-left: w13 -> [w478]
    tunnel: w17 -> [_]
    tunnel: w15 -> [w472]
    shift-right: [w471] -> _
    shift-left: w16 -> [w474]
    stop <- w476 stop-if-true
    # "Find And Highlight Loop"
    n196 = Wait Until Next ms Multiple(millisecond multiple=u32 50) -> ()  [unwired: 1 out]
    n197 = local read "Exit"() -> (w475:bool)
    n198 = case shown="False" w475 {
      selector: w475 -> [_ w498]
      tunnel: w473 -> [_ _]
      tunnel: w480 -> [w485 _]
      tunnel: w474 -> [w488 w496]
      tunnel: [w492 w497] -> w479
      tunnel: w478 -> [w486 w497]
      tunnel: [_ w498] -> w476
      tunnel: w472 -> [w491 _]
      tunnel: [w487 w496] -> w471
      frame False {
        n199 = Wait on Notification(notifier=w485, error in (no error)=w486) -> (notifier out=w481:refnum<notifier>, notification=w482:cluster{"X":i32, "Y":i32}, error out=w484:errorcluster)  [unwired: 2 in, 1 out]
        n200 = Cancel Notification(0:w481, 3:w484) -> (11:w483:errorcluster)  [unwired: 2 out]
        n201 = Unbundle(w482) -> ("X"=w494:i32, "Y"=w495:i32)
        n202 = local read "Points"() -> (w493:i32[][])
        n203 = call "FindAndHighlightPoint.vi"("Data In"=w488, "error in (no error)"=w483, "Vertical"=w495, "Horizontal"=w494, "Value"=w493) -> ("error out"=w492:errorcluster, "Data Out"=w487:T1)  [unwired: 4 in, 1 out]
        n204 = To Variant(anything=w487) -> (Variant=w489:variant)
        n205 = call-poly "Enqueue Message.vi"("Message Data"=w489, "Message"="Sync Settings", "Message Queue"=w491) -> ()  [unwired: 7 in, 2 out]
      }
      frame True {
      }
    }
  }
  n206 = Unregister For Events(event registration refnum=w21) -> ()  [unwired: 1 in, 1 out]
